vi "Jenkins - Get Console Text.vi"(8 "error in (no error)":errorcluster, 10 "Script Job Name (Within Build Script Folder)":string, 11 "IP Address":string) -> (0 "error out":errorcluster, 3 "Text":string)   [LabVIEW 2014]
uses:
  <vilib>/httpClient/LabVIEWHTTPClient.lvlib
  <vilib>/wsapi/NI_WebServices.lvlib
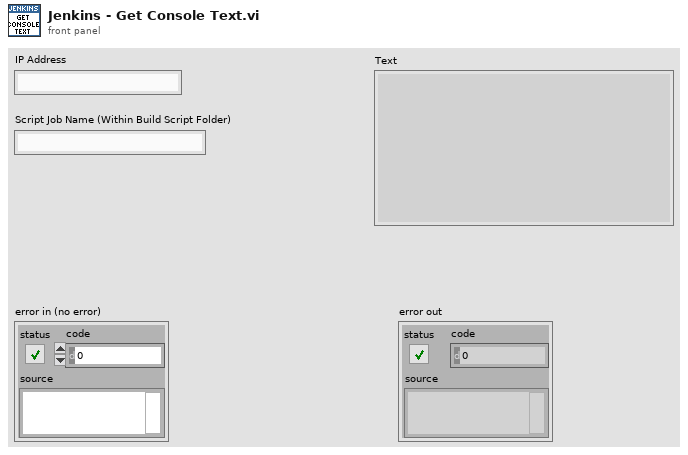
[diagram p1: front panel]
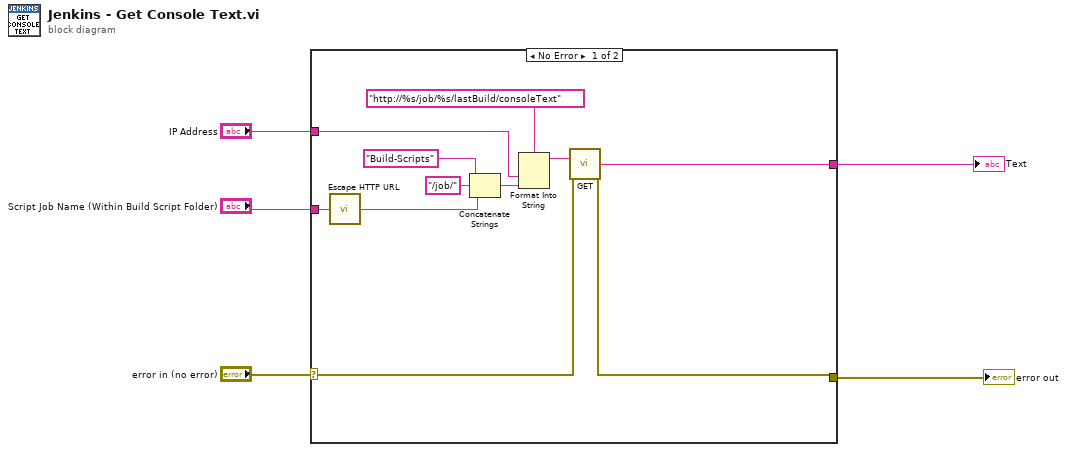
[diagram p0: block diagram]
diagram:
  n1 = case shown="No Error" "error in (no error)" {
    selector: "error in (no error)" -> [w8 w17]
    tunnel: "IP Address" -> [w11 _]
    tunnel: "Script Job Name (Within Build Script Folder)" -> [w10 _]
    tunnel: [w6 w17] -> w3
    tunnel: [w7 _] -> w1
    frame No Error {
      n2 = call <vilib>:"Escape HTTP URL.vi"("unescaped string in"=w10) -> ("escaped string out"=w9:string)
      n3 = Concatenate Strings("Build-Scripts" ("JSON"), "/job/" ("string"), w9) -> (w12:string)
      n4 = Format Into String(format string="http://%s/job/%s/lastBuild/consoleText", w11, w12) -> (resulting string=w16:string)  [unwired: 2 in, 1 out]
      n5 = call <vilib>:"GET.vi"("url"=w16, "error in (no error)"=w8) -> ("body"=w7:string, "error out"=w6:errorcluster)  [unwired: 10 in, 2 out]
    }
    frame Error {
    }
  }
  "error out" <- w3
  "Text" <- w1
